vi "CoreAudioGenerator.vi"(11 "Cluster":T1) -> ()   [LabVIEW 2024]
uses:
  #PlayLoopEnum.ctl
  <vilib>/sound2/lvsound2.llb/Sampling Mode.ctl
  GUI/#GuiEnum.ctl
  GUI/#GuiQueueElement.ctl
  <vilib>/sound2/lvsound2.llb/Sound Output Write (DBL Single).vi
  <vilib>/sound2/lvsound2.llb/Sound Output Task ID.ctl
  <vilib>/vision/Image Controls.llb/IMAQ Image.ctl
  vision/#QueueEnum.ctl
  Core/#CoreQueues.ctl
  Correlation/#CorrelationQueueElement.ctl
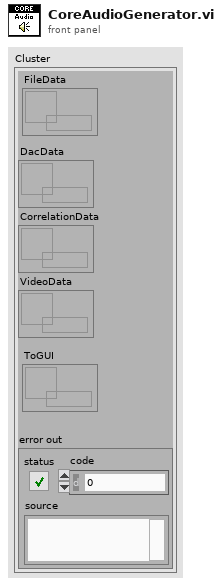
[diagram p1: front panel]
types:
  T1 = typedef "#CoreQueues.ctl" = cluster{"DacData":refnum<queue>, "CorrelationData":refnum<queue>, "VideoData":refnum<queue>, "error out":errorcluster, "ToGUI":refnum<queue>, "FileData":refnum<queue>}
  T2 = typedef "#PlayLoopEnum.ctl" = enum16{"Idle", "Init", "Play", "End"}
  T3 = typedef "#GuiEnum.ctl" = enum16{"AudioData", "VisionDistances", "DacDistances", "CorrelationDistances", "Video", "FPS"}
  T4 = typedef "#GuiQueueElement.ctl" = cluster{"Enum":T3, "Variant":variant}
  T5 = typedef "Sound Output Task ID.ctl" = u32
  T6 = typedef "Sampling Mode.ctl" = i32
  T7 = typedef "#AquisitionParameter.ctl" = cluster{"SampleRate":dbl, "BufferSize":i32, "Channels":tag}
  T8 = typedef "Sound Data Format.ctl" = cluster{"sample rate (S/s)":dbl, "number of channels":i32, "bits per sample":i32}
  T9 = cluster{"AquisitionParameters":T7, "SoundFormat":T8, "Signal type":enum16{"Sine Wave", "Triangle Wave", "Square Wave", "Sawtooth Wave"}, "Amplitude":dbl, "AudioBuffer":i32, "ChannelBounds":cluster{"InputMin":dbl, "InputMax":dbl, "OutputMin":dbl, "OutputMax":dbl}[], "MasterOffset":dbl}
  T10 = enum16{"Sine Wave", "Triangle Wave", "Square Wave", "Sawtooth Wave"}
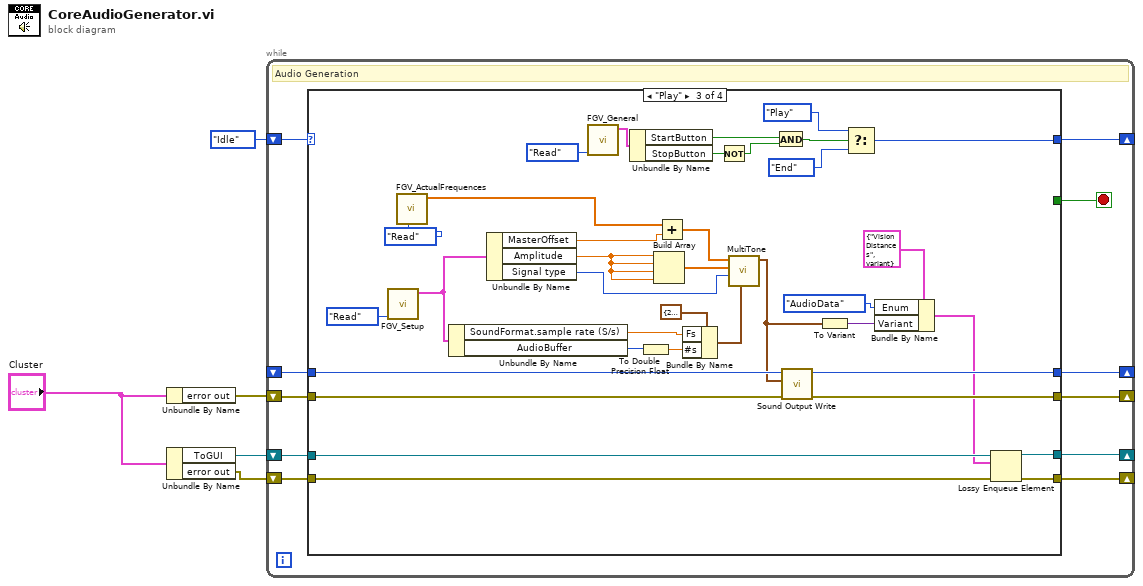
[diagram p0: block diagram]
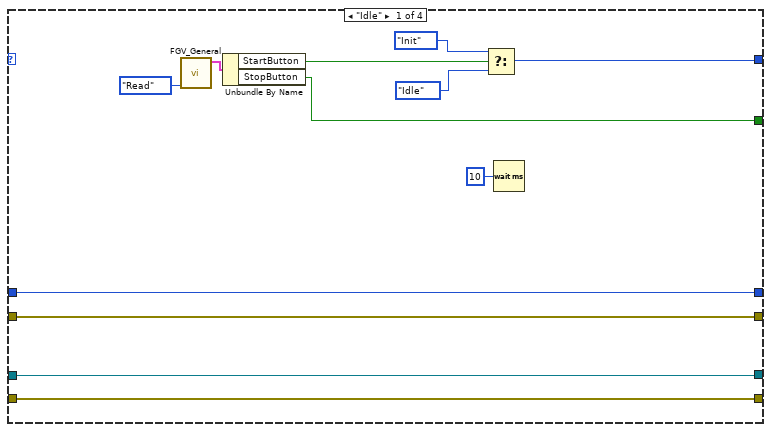
[diagram p2: hidden frame]
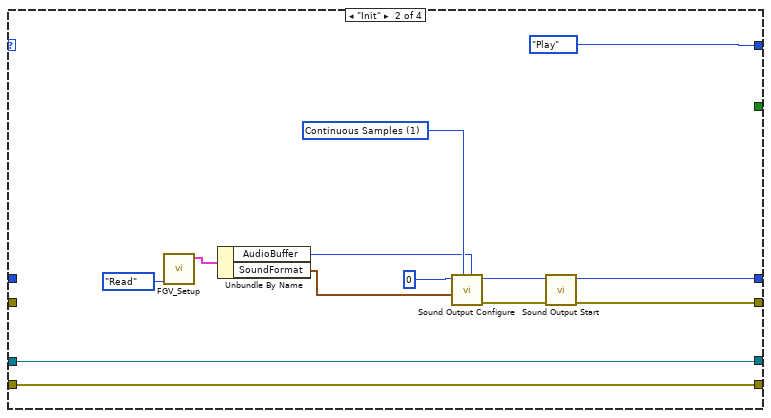
[diagram p3: hidden frame]
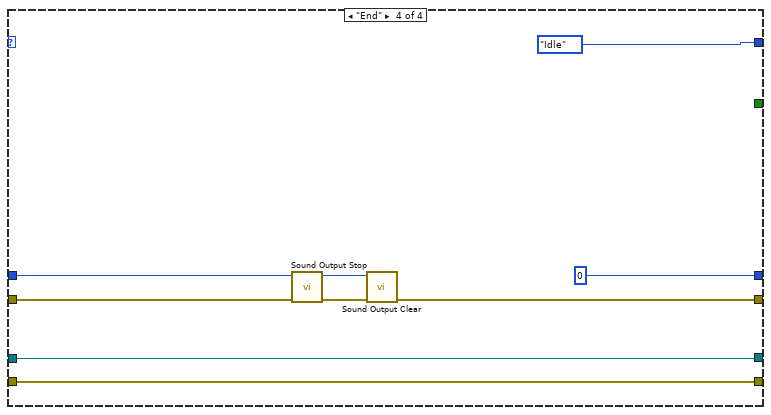
[diagram p4: hidden frame]
diagram:
  n1 = Unbundle By Name("Cluster") -> ("error out"=w2:errorcluster)
  n2 = Unbundle By Name("Cluster") -> ("ToGUI"=w4:refnum<queue>, "error out"=w5:errorcluster)
  n3 = while {
    shift-right: [w13] -> _
    shift-left: _ -> [w16]
    shift-right: [w14] -> _
    shift-left: w2 -> [w15]
    shift-right: [w11] -> _
    shift-left: #PlayLoopEnum."Idle" -> [w12]
    shift-right: [w8] -> _
    shift-left: w4 -> [w9]
    shift-right: [w6] -> _
    shift-left: w5 -> [w7]
    stop <- w10 stop-if-true
    # "Audio Generation"
    n4 = case shown="\"Play\"" w12 {
      tunnel: w16 -> [w25 _ w77 w84]
      tunnel: w15 -> [w19 _ w76 w83]
      tunnel: [w19 w36 w75 w82] -> w14
      tunnel: [w25 w37 w74 T5 0 ("task ID out")] -> w13
      tunnel: [w27 #PlayLoopEnum."Play" w73 #PlayLoopEnum."Idle"] -> w11
      tunnel: [w21 _ _ _] -> w10
      tunnel: w9 -> [w18 w30 w50 w79]
      tunnel: [w18 w30 w49 w79] -> w8
      tunnel: w7 -> [w17 w29 w48 w78]
      tunnel: [w17 w29 w47 w78] -> w6
      frame "Idle" {
        n5 = call "FGV_General.vi"("Type"=enum16{"Read", "Write"}."Read") -> ("GeneralIndicator"=w22:cluster{"StartButton":bool, "StopButton":bool})  [unwired: 10 in]
        n6 = Unbundle By Name(w22) -> ("StartButton"=w20:bool, "StopButton"=w21:bool)
        n7 = Select(t=#PlayLoopEnum."Init", s=w20, f=#PlayLoopEnum."Idle") -> (s? t:f=w27:T2)
        n8 = Wait (ms)(milliseconds to wait=u32 10) -> ()  [unwired: 1 out]
      }
      frame "Init" {
        w39 = T6 1 items=["Finite Samples", "Continuous Samples"] ("sample mode")
        n9 = call "FGV_Setup.vi"("Type"=enum16{"Read", "Write"}."Read") -> ("OutSetup"=w33:T9)  [unwired: 10 in]
        n10 = Unbundle By Name(w33) -> ("AudioBuffer"=w31:i32, "SoundFormat"=w32:T8)
        n11 = call <vilib>:"Sound Output Configure.vi"("number of samples/ch"=w31, "sample mode"=w39, "sound format"=w32, "device ID"=u32 0) -> ("error out"=w41:errorcluster, "task ID"=w40:T5)  [unwired: 6 in]
        n12 = call <vilib>:"Sound Output Start.vi"("error in (no error)"=w41, "task ID"=w40) -> ("error out"=w36:errorcluster, "task ID out"=w37:T5)  [unwired: 8 in]
      }
      frame "Play" {
        n13 = call "FGV_Setup.vi"("Type"=enum16{"Read", "Write"}."Read") -> ("OutSetup"=w54:T9)  [unwired: 10 in]
        n14 = call "FGV_ActualFrequences.vi"("Type"=enum16{"Read", "Write"}."Read") -> ("Frequences"=w52:dbl[])  [unwired: 10 in]
        n15 = Unbundle By Name(w54) -> ("SoundFormat.sample rate (S/s)"=w68:dbl, "AudioBuffer"=w58:i32)
        n16 = Unbundle By Name(w54) -> ("MasterOffset"=w53:dbl, "Amplitude"=w59:dbl, "Signal type"=w60:T10)
        n17 = call "FGV_General.vi"("Type"=enum16{"Read", "Write"}."Read") -> ("GeneralIndicator"=w65:cluster{"StartButton":bool, "StopButton":bool})  [unwired: 10 in]
        n18 = Unbundle By Name(w65) -> ("StartButton"=w63:bool, "StopButton"=w64:bool)
        n19 = To Double Precision Float(number=w58) -> (double precision float=w57:dbl)
        n20 = Build Array(w59, w59, w59, w59) -> (w67:dbl[])
        n21 = Add(x=w52, y=w53) -> (x+y=w61:dbl[])
        n22 = Bundle By Name(cluster=cluster{"Fs":dbl, "#s":dbl} {"Fs"=22050.0, "#s"=0.0} ("Sampling Info"), "Fs"=w68, "#s"=w57) -> (w55:cluster{"Fs":dbl, "#s":dbl})
        n23 = Not(x=w64) -> (.not. x?=w69:bool)
        n24 = call "MultiTone.vi"("Sampling Info"=w55, "Signal type"=w60, "Amplitudes"=w67, "Frequences"=w61) -> ("Output"=w43:waveform(dbl))  [unwired: 7 in]
        n25 = And(x=w63, y=w69) -> (x .and. y?=w70:bool)
        n26 = call-poly <vilib>:"Sound Output Write.vi"("error in (no error)"=w76, "data"=w43, "task ID"=w77) -> ("error out"=w75:errorcluster, "task ID out"=w74:T5)  [unwired: 7 in]
        n27 = To Variant(anything=w43) -> (Variant=w45:variant)
        n28 = Select(t=#PlayLoopEnum."Play", s=w70, f=#PlayLoopEnum."End") -> (s? t:f=w73:T2)
        n29 = Bundle By Name(cluster=T4 {"Enum"=enum."VisionDistances", "Variant"=variant} ("element"), "Enum"=#GuiEnum."AudioData", "Variant"=w45) -> (w42:T4)
        n30 = Lossy Enqueue Element(queue=w50, element=w42, error in (no error)=w48) -> (queue out=w49:refnum<queue>, error out=w47:errorcluster)  [unwired: 2 out]
      }
      frame "End" {
        n31 = call <vilib>:"Sound Output Stop.vi"("error in (no error)"=w83, "task ID"=w84) -> ("error out"=w86:errorcluster, "task ID out"=w85:T5)  [unwired: 8 in]
        n32 = call <vilib>:"Sound Output Clear.vi"("error in (no error)"=w86, "task ID"=w85) -> ("error out"=w82:errorcluster)  [unwired: 9 in]
      }
    }
  }
